vi "Open Configuration Reference.vi"(8 "error in (no error)":errorcluster, 11 "Configuration Type":refnum<class "IConfiguration.lvclass">) -> (0 "error out":errorcluster, 3 "Configuration Reference":refnum<data-value>)   [LabVIEW 2017, in "Configuration.lvlib" / "ConfigurationReference.lvclass"]
uses:
  ConfigurationReference.lvclass
  IConfiguration/IConfiguration.lvclass
  ConfigurationReference.lvclass/ConfigurationReference.ctl
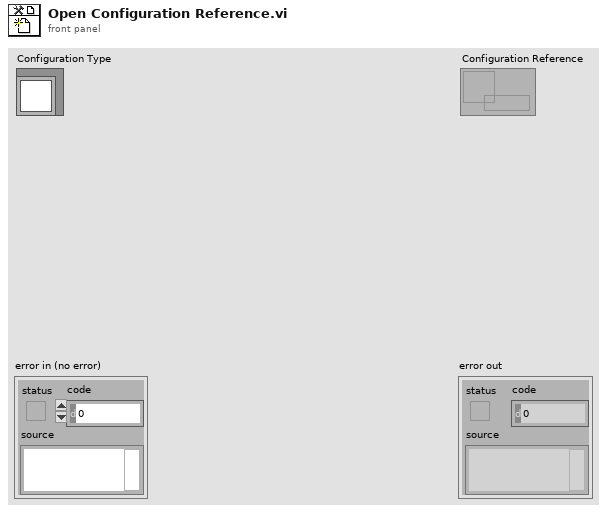
[diagram p1: front panel]
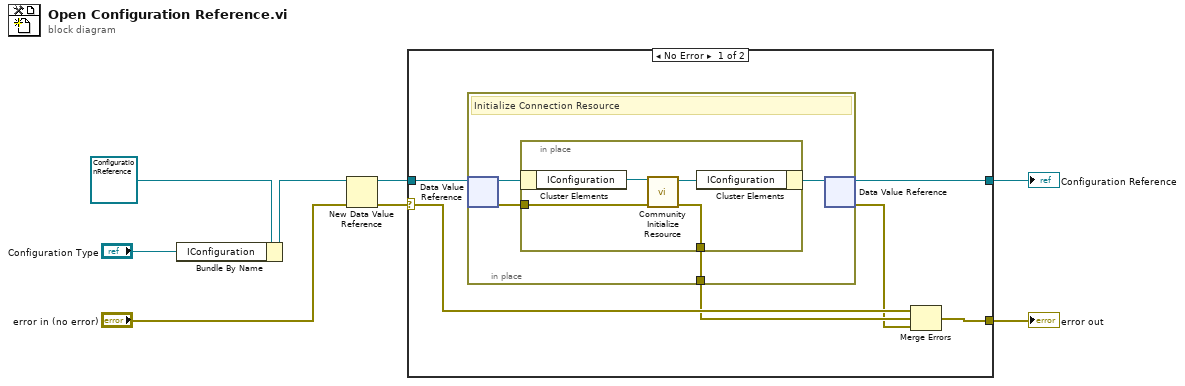
[diagram p0: block diagram]
diagram:
  n1 = Bundle By Name(cluster=refnum<class "ConfigurationReference.lvclass"> refnum ("ConfigurationReference out"), "IConfiguration"="Configuration Type") -> (w5:refnum<class "ConfigurationReference.lvclass">)
  n2 = New Data Value Reference(data value=w5, error in="error in (no error)") -> (data value reference=w4:refnum<data-value>, error out=w2:errorcluster)
  n3 = case shown="No Error" w2 {
    selector: w2 -> [w11 w23]
    tunnel: w4 -> [w14 w24]
    tunnel: [w13 w24] -> w3
    tunnel: [w12 w23] -> w1
    frame No Error {
      n4 = in-place {
        in-place-border: [w16] -> w10
        # "Initialize Connection Resource"
        n5 = in-place-dvr #1(w14) -> (w18:refnum<class "ConfigurationReference.lvclass">, w15:errorcluster)
        n6 = in-place {
          in-place-border: [w20] -> w16
          in-place-border: w15 -> [w19]
          n7 = in-place-cluster #2(w18) -> ("IConfiguration"=w22:refnum<class "IConfiguration.lvclass">)
          n8 = call "Community Initialize Resource.vi"("error in (no error)"=w19, "IConfiguration in"=w22) -> ("error out"=w20:errorcluster, "IConfiguration out"=w21:refnum<class "IConfiguration.lvclass">)  [unwired: 8 in]
          n9 = in-place-cluster #2("IConfiguration"=w21) -> (w17:refnum<class "ConfigurationReference.lvclass">)
        }
        n10 = in-place-dvr #1(w17) -> (w13:refnum<data-value>, w9:errorcluster)
      }
      n11 = Merge Errors(w11, w10, w9) -> (w12:errorcluster)
    }
    frame Error {
    }
  }
  "error out" <- w1
  "Configuration Reference" <- w3
